vi "Default Config Settings.vi"(8 "error in (no error)":errorcluster) -> (0 "error out":errorcluster, 2 "Config Settings":T1={"Application Settings"={"Simulation"=FALSE}, "Main Settings"={"Simulation"=FALSE, "Signal scaling"=[], "ESR scaling"=[], "num readings to average"=[], "ESR alarm threshhold (%)"=[], "UseDummyVrms"=FALSE, "Dummy Vrms"=0.0, "Inverter Database File"=path "", "default Inverter (name)"=[]}, "DAQ Settings"={"Simulation"=FALSE, "Initial ErrReporting setting"=0, "Initial Measurement settings"={"Data Rate 9775"=20.0, "Data Rate 9215"=20.0, "Samples RMS 9215"=1000, "Samples RMS 9775"=1000}, "Acquisition mode"=enum."3phase", "DemoMode"=FALSE, "RIO Device"=""}, "LogEngine Settings"={"Simulation"=FALSE, "TDMS_FolderPath"="", "CSV_FolderPath"="", "TDMS_FileName_Prefix"="", "CSV_FileName_Prefix"="", "TDMS_LogDuration(s)"=0.0, "CSV_LogDuration(s)"=0.0}} {"Main Settings"."Dummy Vrms" format="%.2g"; "DAQ Settings"."Initial ErrReporting setting" items=["DONTPRINT", "PRINTWARNINGS", "PRINTFATAL", "PRINTALL"]})   [LabVIEW 2019, in "Config.lvclass"]
doc: "Developed by Kevin Thompson\nkevin@thompsonengineering.net\n\nCopyright 2018-2020\nThompson Engineering, LLC"
uses:
  Config.lvclass
  DataTypes/Config Settings.ctl
  Application/DataTypes/Settings--cluster.ctl
  Main/DataTypes/Settings--cluster.ctl
  Main/support/Data Algorithms/subvis/DataTypes/Gain control.ctl
  Main/support/Data Algorithms/subvis/DataTypes/ESR scaling--cluster.ctl
  DAQ_Engine/DataTypes/Settings--cluster.ctl
  Common/DataTypes/Measurement Config--cluster.ctl
  Common/DataTypes/Acquisition Mode--cluster.ctl
  Log_Engine/DataTypes/Settings--cluster.ctl
  Application/Application.lvclass
  Log_Engine/Log_Engine.lvclass
  DAQ_Engine/DAQ_Engine.lvclass
  Main/Main.lvclass
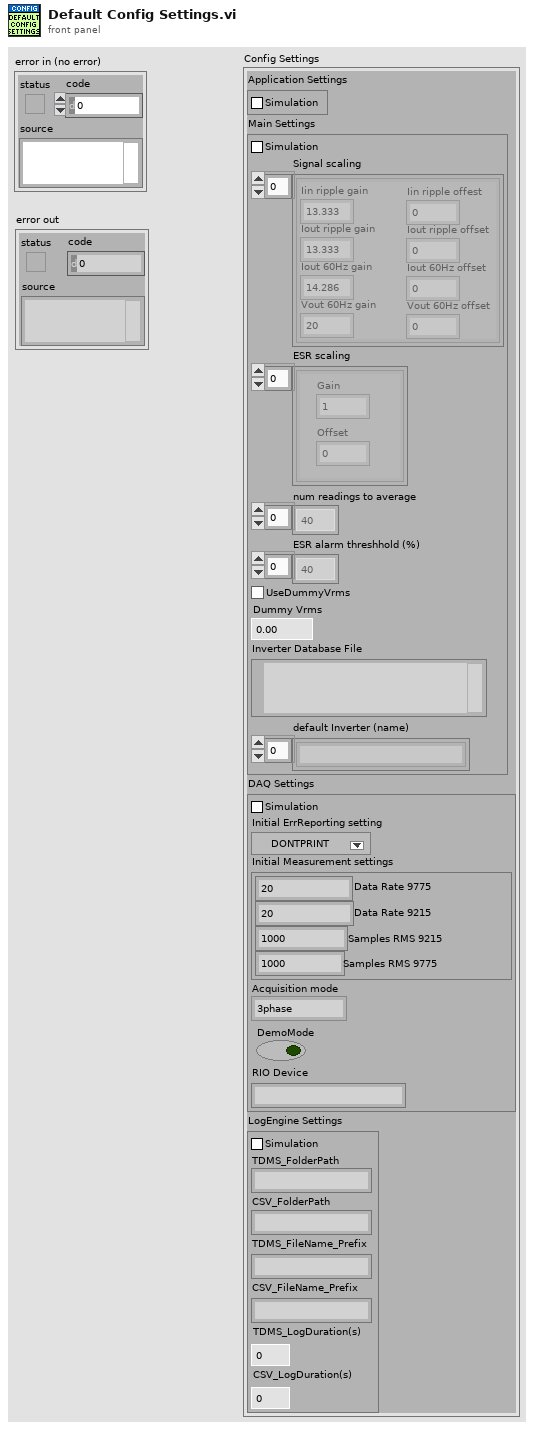
[diagram p1: front panel]
types:
  T1 = typedef "Config.lvclass/Config Settings.ctl" = cluster{"Application Settings":T2, "Main Settings":T3, "DAQ Settings":T6, "LogEngine Settings":T9}
  T2 = typedef "Application.lvclass/Settings--cluster.ctl" = cluster{"Simulation":bool}
  T3 = typedef "Main.lvclass/Settings--cluster.ctl" = cluster{"Simulation":bool, "Signal scaling":T4[], "ESR scaling":T5[], "num readings to average":i32[], "ESR alarm threshhold (%)":i32[], "UseDummyVrms":bool, "Dummy Vrms":dbl, "Inverter Database File":path, "default Inverter (name)":string[]}
  T4 = typedef "Main.lvclass/Gain control.ctl" = cluster{"Iin ripple gain":dbl, "Iout ripple gain":dbl, "Iout 60Hz gain ":dbl, "Vout 60Hz gain ":dbl, "Iin ripple offest":dbl, "Iout ripple offset":dbl, "Iout 60Hz offset":dbl, "Vout 60Hz offset":dbl}
  T5 = typedef "Main.lvclass/ESR scaling--cluster.ctl" = cluster{"Gain":dbl, "Offset":dbl}
  T6 = typedef "DAQ_Engine.lvclass/Settings--cluster.ctl" = cluster{"Simulation":bool, "Initial ErrReporting setting":i32, "Initial Measurement settings":T7, "Acquisition mode":T8, "DemoMode":bool, "RIO Device":string}
  T7 = typedef "Measurement Config--cluster.ctl" = cluster{"Data Rate 9775":dbl, "Data Rate 9215":dbl, "Samples RMS 9215":u32, "Samples RMS 9775":u32}
  T8 = typedef "Acquisition Mode--cluster.ctl" = enum16{"3phase", "Single"}
  T9 = typedef "Log_Engine.lvclass/Settings--cluster.ctl" = cluster{"Simulation":bool, "TDMS_FolderPath":string, "CSV_FolderPath":string, "TDMS_FileName_Prefix":string, "CSV_FileName_Prefix":string, "TDMS_LogDuration(s)":dbl, "CSV_LogDuration(s)":dbl}
  T10 = cluster{"Simulation":bool, "TDMS_FolderPath":string, "CSV_FolderPath":string, "TDMS_FileName_Prefix":string, "CSV_FileName_Prefix":string, "TDMS_LogDuration(s)":dbl, "CSV_LogDuration(s)":dbl}
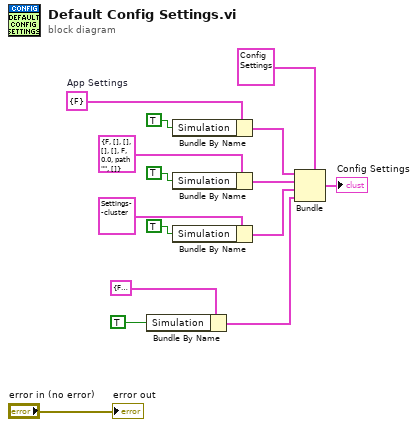
[diagram p0: block diagram]
diagram:
  w14 = T2 {"Simulation"=FALSE}  # App Settings
  n1 = Bundle By Name(cluster=T10 {"Simulation"=FALSE, "TDMS_FolderPath"="", "CSV_FolderPath"="", "TDMS_FileName_Prefix"="", "CSV_FileName_Prefix"="", "TDMS_LogDuration(s)"=0.0, "CSV_LogDuration(s)"=0.0} ("Settings"), "Simulation"=TRUE) -> (w6:T10)
  n2 = Bundle By Name(cluster=w14, "Simulation"=TRUE) -> (w13:T2)
  n3 = Bundle By Name(cluster=T3 {"Simulation"=FALSE, "Signal scaling"=[], "ESR scaling"=[], "num readings to average"=[], "ESR alarm threshhold (%)"=[], "UseDummyVrms"=FALSE, "Dummy Vrms"=0.0, "Inverter Database File"=path "", "default Inverter (name)"=[]} ("Settings"), "Simulation"=TRUE) -> (w8:T3)
  n4 = Bundle By Name(cluster=T6 {"Simulation"=FALSE, "Initial ErrReporting setting"=0, "Initial Measurement settings"={"Data Rate 9775"=1000000.0, "Data Rate 9215"=20000.0, "Samples RMS 9215"=1000, "Samples RMS 9775"=10000}, "Acquisition mode"=enum."Single", "DemoMode"=FALSE, "RIO Device"=""} ("Settings"), "Simulation"=TRUE) -> (w7:T6)
  n5 = Bundle(cluster=T1 {"Application Settings"={"Simulation"=FALSE}, "Main Settings"={"Simulation"=FALSE, "Signal scaling"=[], "ESR scaling"=[], "num readings to average"=[], "ESR alarm threshhold (%)"=[], "UseDummyVrms"=FALSE, "Dummy Vrms"=0.0, "Inverter Database File"=path "", "default Inverter (name)"=[]}, "DAQ Settings"={"Simulation"=FALSE, "Initial ErrReporting setting"=0, "Initial Measurement settings"={"Data Rate 9775"=20.0, "Data Rate 9215"=20.0, "Samples RMS 9215"=1000, "Samples RMS 9775"=1000}, "Acquisition mode"=enum."3phase", "DemoMode"=FALSE, "RIO Device"=""}, "LogEngine Settings"={"Simulation"=FALSE, "TDMS_FolderPath"="", "CSV_FolderPath"="", "TDMS_FileName_Prefix"="", "CSV_FileName_Prefix"="", "TDMS_LogDuration(s)"=0.0, "CSV_LogDuration(s)"=0.0}} ("Config Settings"), "Application Settings"=w13, "Main Settings"=w8, "DAQ Settings"=w7, "LogEngine Settings"=w6) -> (→"Config Settings":T1)
  "error out" <- "error in (no error)"
